vi "AnalogCNTL.vi"() -> ()   [LabVIEW 2015]
panel:
  out "Numeric 2":dbl
  in  "Knob 2":dbl(knob) min=0.0 max=5.0 step=0.01 scale=0.0..5.0
  out "Numeric":dbl
  in  "Knob":dbl(knob) min=0.0 max=5.0 step=0.01 scale=0.0..5.0
  in  "stop":bool
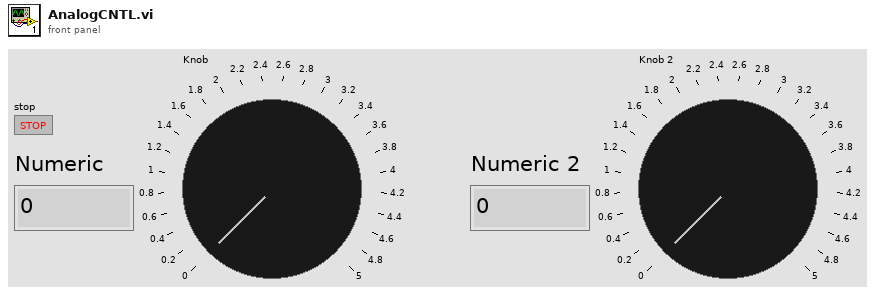
[diagram p1: front panel]
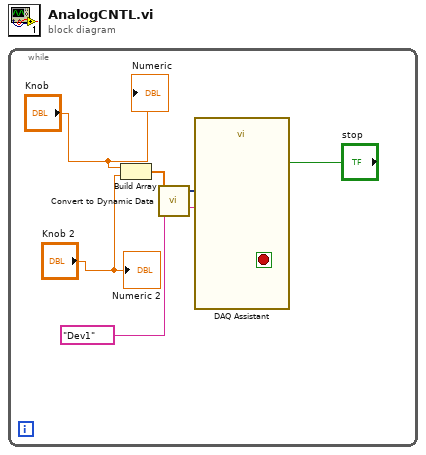
[diagram p0: block diagram]
diagram:
  n1 = while {
    stop <- "stop" stop-if-true
    n2 = Build Array("Knob", "Knob 2") -> (w4:dbl[])
    n3 = call "Convert to Dynamic Data"("Array"=w4) -> ("Dynamic Data Type"=w2:dynamicdata)  [unwired: 3 in]
    n4 = call "DAQ Assistant"("data"=w2, "device name"=tag "Dev1") -> ()  [unwired: 16 in, 2 out]
    "Numeric" <- "Knob"
    "Numeric 2" <- "Knob 2"
  }
